vi "main 2nd.vi"() -> ()   [LabVIEW 2015]
uses:
  <vilib>/Utility/file.llb/Read From Spreadsheet File (DBL).vi
panel:
  out "From OD fit?":bool
  out "Current file num":i32
  out "ROI Width":u32
  out "ROI Height":u32
  in  "Image Dark":dbl[][](array[numeric])
  in  "Image Light":dbl[][](array[numeric])
  in  "Image Atom":dbl[][](array[numeric])
  out "Best fit parameters":dbl[](array[numeric])
  out "Fitting Results Save Path":string[](array[string])
  out "Best fit results":dbl[][](array[numeric])
  in  "Initial guess values":dbl[](array[numeric])
  in  "Latest image data":dbl[][](array[numeric])
  out "Fitting Type":u16(ring)
  out "Force Guess?":bool
  out "Aquired?":bool
  out "Process Index":i32
  out "External Trigger":bool
  out "XY图":cluster{dbl[], dbl[]}[](graph)
  out "OD Image":dbl[][](graph)
  in  "OD fit":bool
  in  "OD num":i32
  out "Fit Done":bool
  in  "Exit":bool
  out "XY图 2":cluster{dbl[], dbl[]}[](graph)
  in  "Auto Split":bool
  in  "Fit":bool
  in  "Open File":bool
  in  "Auto Fit":bool
  in  "Stop":bool
  in  "Aquire":bool
  in  "Fitting Config":bool
  in  "Camera Config":bool
  in  "Initialize":bool
  in  "Live Image Display":refnum<k7>(container)
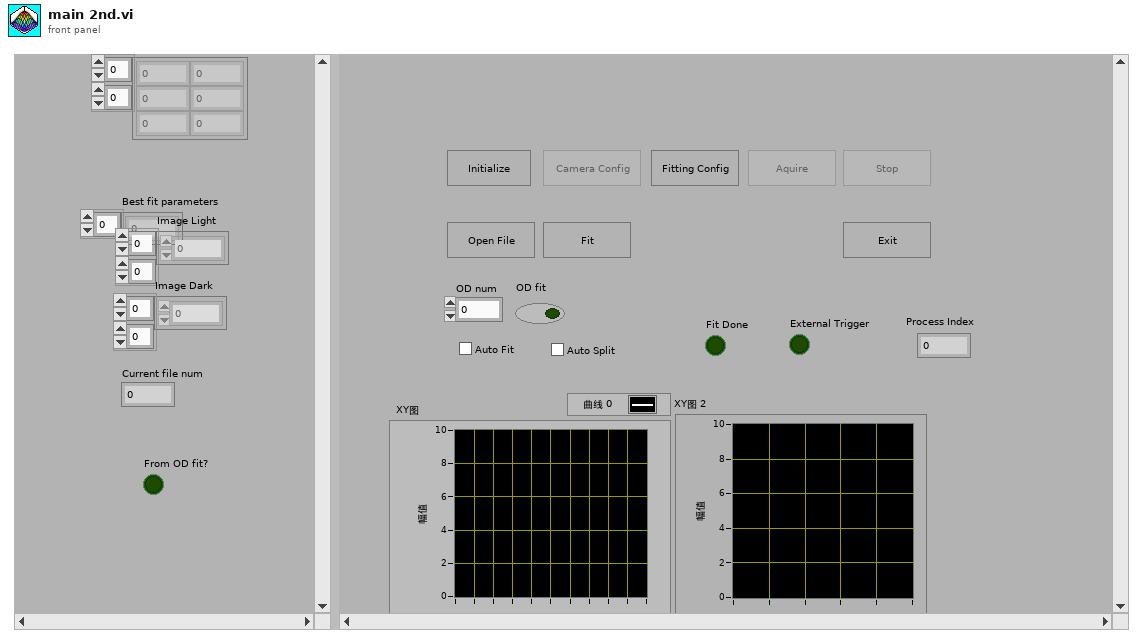
[diagram p1: front panel]
types:
  T1 = enum8{"Enabled", "Disabled", "Disabled and Grayed Out"}
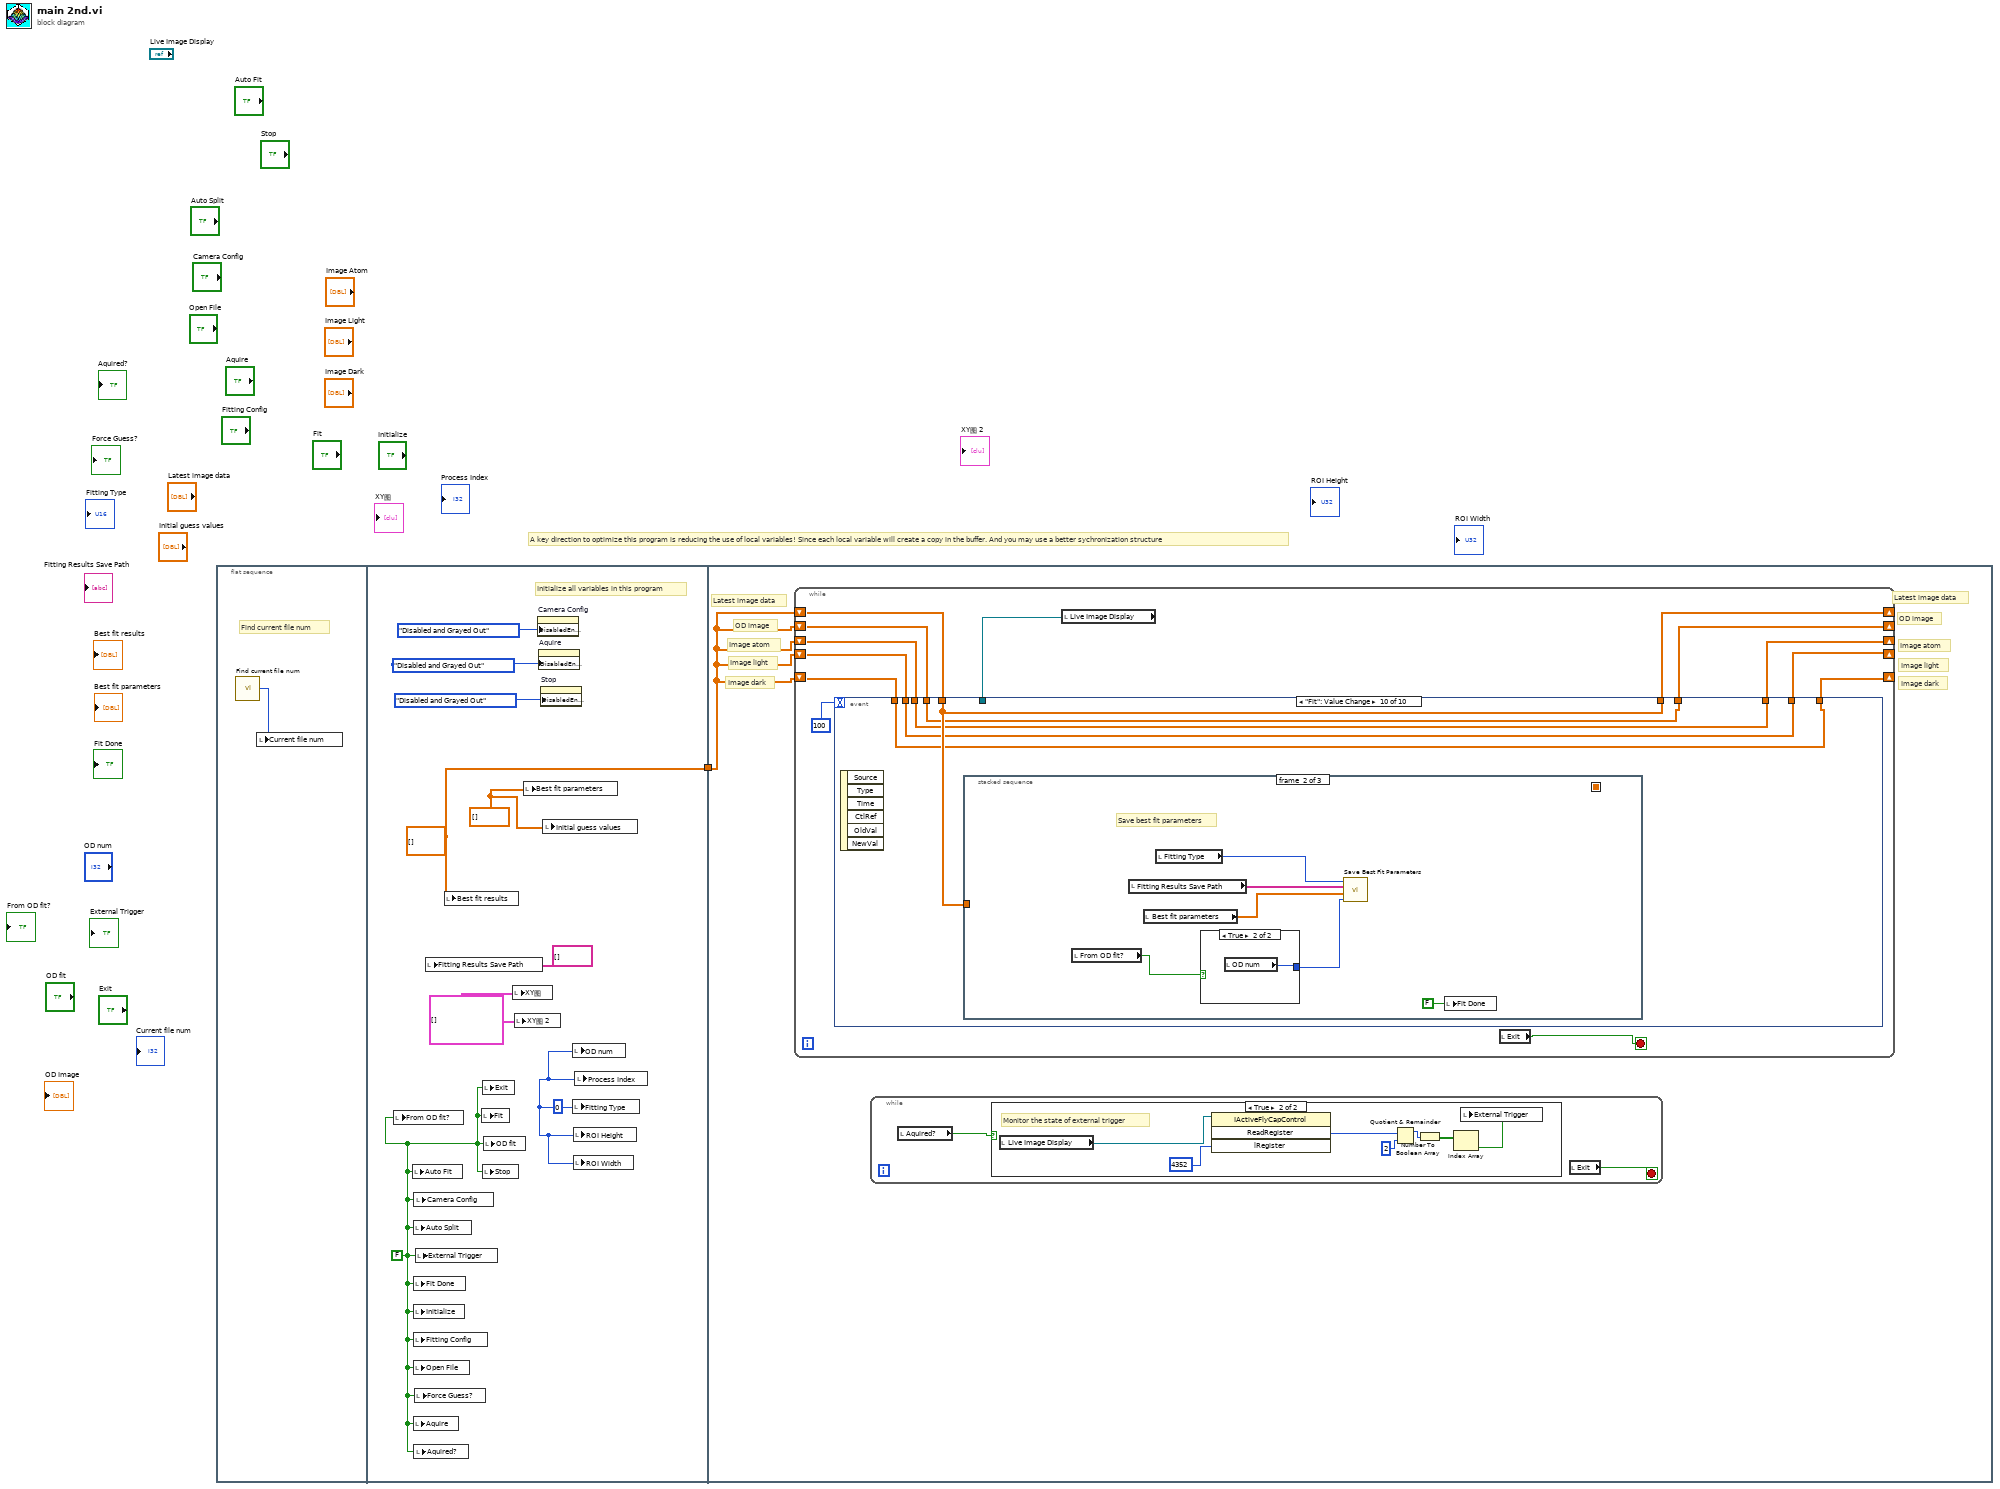
[diagram p0: block diagram]
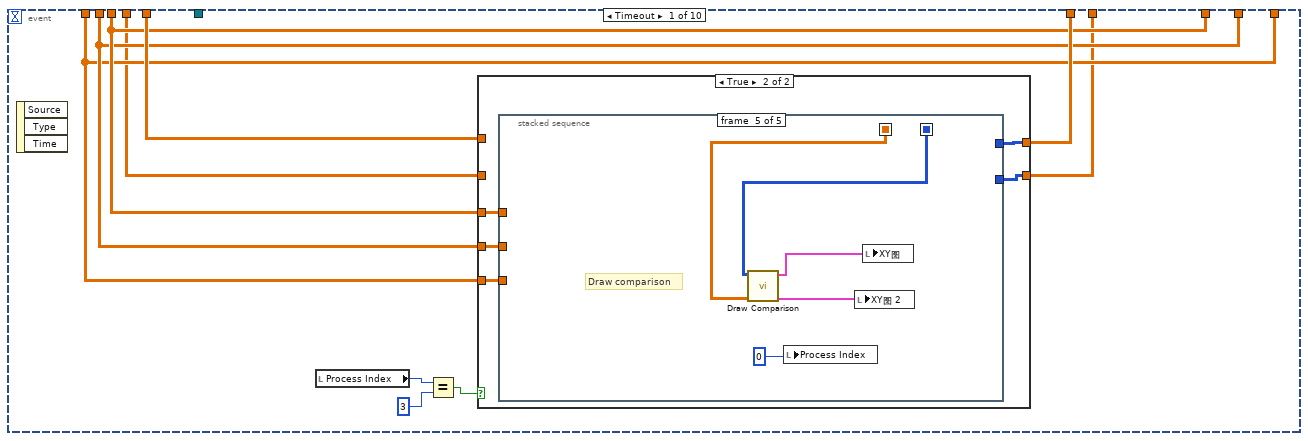
[diagram p3: hidden frame]
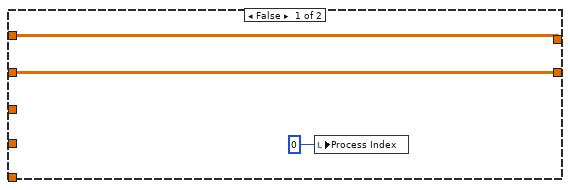
[diagram p4: hidden frame]
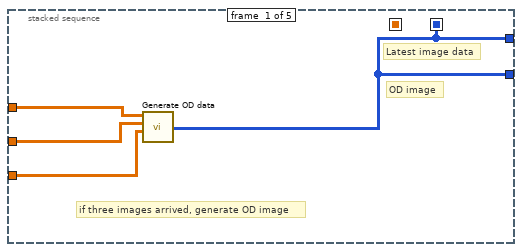
[diagram p5: hidden frame]
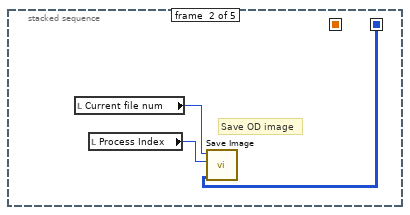
[diagram p6: hidden frame]
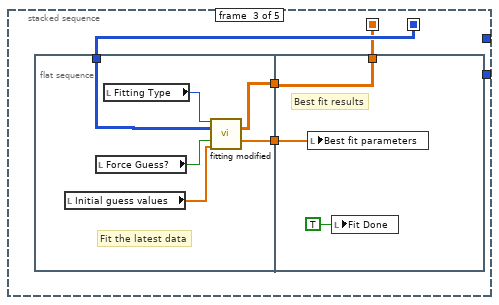
[diagram p7: hidden frame]
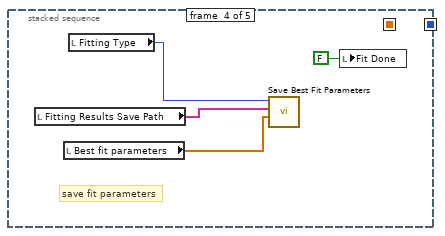
[diagram p8: hidden frame]
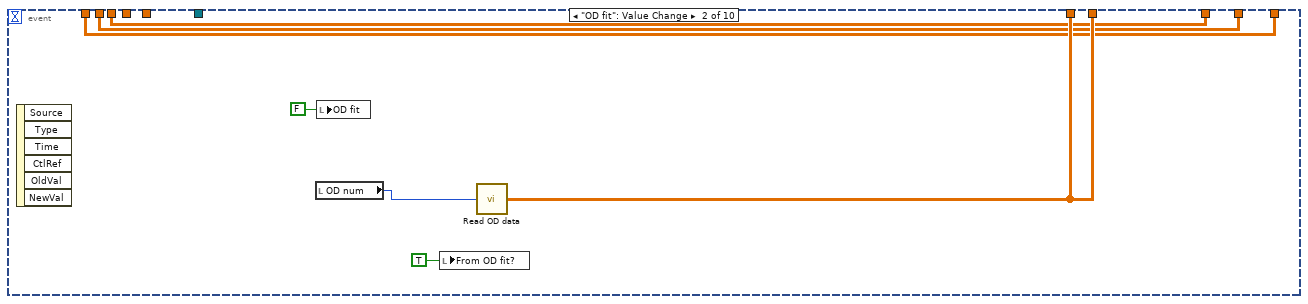
[diagram p9: hidden frame]
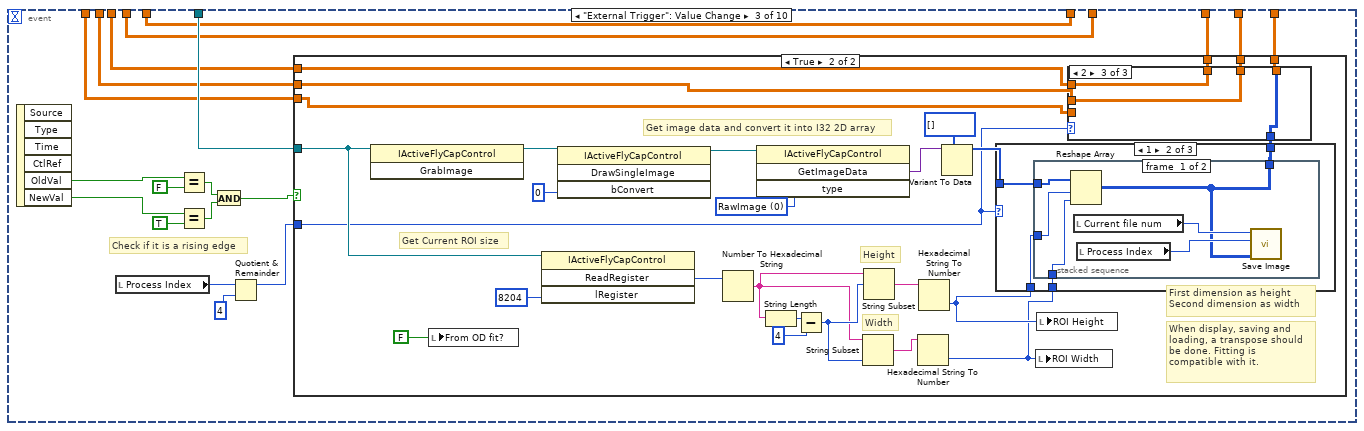
[diagram p10: hidden frame]
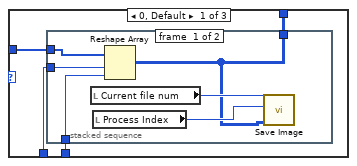
[diagram p14: hidden frame]
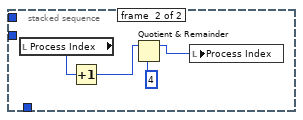
[diagram p15: hidden frame]
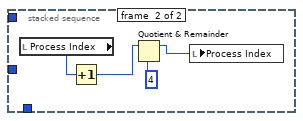
[diagram p16: hidden frame]
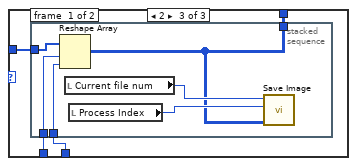
[diagram p17: hidden frame]
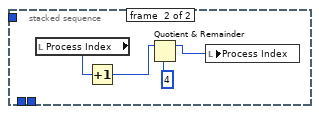
[diagram p18: hidden frame]
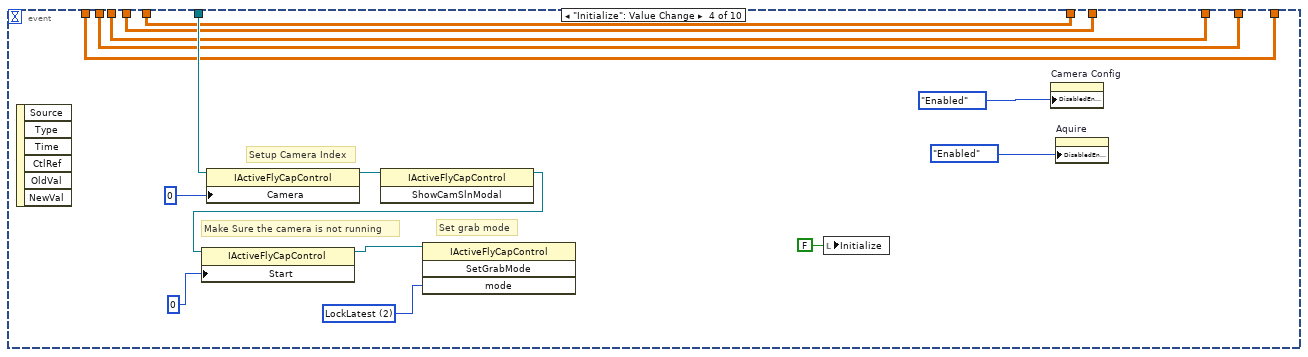
[diagram p19: hidden frame]
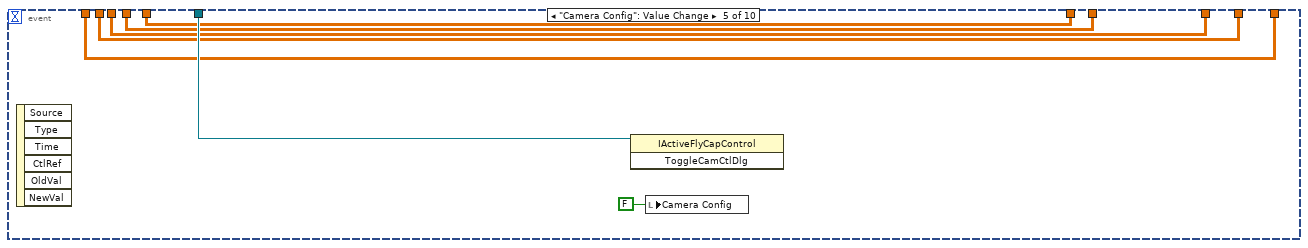
[diagram p20: hidden frame]
diagram:
  # "A key direction to optimize this program is reducing the use of local variables! Since each local variable will create a copy in the buffer. And you may use a better sychronization structure"
  n1 = flat-sequence {
    tunnel: [w5] -> w1
    tunnel: w1 -> [w12]
    frame #0 {
      # "Find current file num"
      n2 = call "Find current file num.vi"() -> ("Current File Num"=w2:u16)  [unwired: 2 in]
      n3 = local write "Current file num"(w2) -> ()
    }
    frame #1 {
      w7 = cluster{dbl[], dbl[]}[] [] ("XY图")
      w6 = 0 ("OD num")
      w5 = dbl[][] [] ("Best fit results")
      w4 = dbl[] [] ("Best fit parameters")
      w3 = FALSE ("Aquire")
      # "Initialize all variables in this program"
      n4 = local write "From OD fit?"(w3) -> ()
      n5 = local write "Auto Fit"(w3) -> ()
      n6 = local write "Auto Split"(w3) -> ()
      n7 = local write "Fit Done"(w3) -> ()
      n8 = local write "Initialize"(w3) -> ()
      n9 = local write "Fitting Config"(w3) -> ()
      n10 = local write "Open File"(w3) -> ()
      n11 = local write "Aquire"(w3) -> ()
      n12 = local write "Camera Config"(w3) -> ()
      n13 = local write "Aquired?"(w3) -> ()
      n14 = local write "Force Guess?"(w3) -> ()
      n15 = local write "External Trigger"(w3) -> ()
      n16 = local write "Fitting Results Save Path"(string[] [] ("Fitting Results Save Path")) -> ()
      n17 = local write "Best fit results"(w5) -> ()
      n18 = local write "Fit"(w3) -> ()
      n19 = local write "Exit"(w3) -> ()
      n20 = local write "Stop"(w3) -> ()
      n21 = local write "OD fit"(w3) -> ()
      n22 = local write "XY图"(w7) -> ()
      n23 = local write "XY图 2"(w7) -> ()
      n24 = local write "Best fit parameters"(w4) -> ()
      n25 = property on="Camera Config" class="Bool (strict)"("DisabledEnum"=T1."Disabled and Grayed Out" ("禁用")) -> ()  [unwired: 2 in, 2 out]
      n26 = property on="Aquire" class="Bool (strict)"("DisabledEnum"=T1."Disabled and Grayed Out" ("禁用")) -> ()  [unwired: 2 in, 2 out]
      n27 = property on="Stop" class="Bool (strict)"("DisabledEnum"=T1."Disabled and Grayed Out" ("禁用")) -> ()  [unwired: 2 in, 2 out]
      n28 = local write "Initial guess values"(w4) -> ()
      n29 = local write "OD num"(w6) -> ()
      n30 = local write "Fitting Type"(w6) -> ()
      n31 = local write "ROI Height"(w6) -> ()
      n32 = local write "ROI Width"(w6) -> ()
      n33 = local write "Process Index"(w6) -> ()
    }
    frame #2 {
      # "Image dark"
      # "Image light"
      # "Image atom"
      # "Image dark"
      # "Image light"
      # "Image atom"
      # "OD image"
      # "Latest image data"
      # "OD image"
      # "Latest image data"
      n34 = while {
        shift-right: [w31] -> _
        shift-left: w12 -> [w30]
        shift-right: [w25] -> _
        shift-left: w12 -> [w22]
        shift-right: [w24] -> _
        shift-left: w12 -> [w28]
        shift-right: [w23] -> _
        shift-left: w12 -> [w27]
        shift-right: [w29] -> _
        shift-left: w12 -> [w26]
        stop <- w32 stop-if-true
        n35 = local read "Live Image Display"() -> (w33:refnum<k7>)
        n36 = event shown="[9] \"Fit\": Value Change" {
          selector: _ -> [_ _ _ _ _ _ _ _ _ _]
          dyn-events: _ -> [_ _ _ _ _ _ _ _ _ _]
          timeout: 100 -> [_ _ _ _ _ _ _ _ _ _]
          tunnel: w33 -> [_ _ w100 w197 w210 _ _ _ _ _]
          tunnel: [w41 w86 w98 w193 w208 w215 w225 w232 w244 w256] -> w31
          tunnel: w30 -> [w40 _ w98 w193 w208 w215 w225 w232 w244 w256]
          tunnel: w22 -> [w36 _ w97 w192 w207 w214 w224 w231 w243 w255]
          tunnel: [w37 w83 w99 w189 w204 w211 w221 w228 w240 w252] -> w29
          tunnel: w28 -> [w39 w85 w96 w191 w206 w213 w223 w230 w242 w254]
          tunnel: w27 -> [w38 w84 w95 w190 w205 w212 w222 w229 w241 w253]
          tunnel: w26 -> [w37 w83 w94 w189 w204 w211 w221 w228 w240 w252]
          tunnel: [w35 w86 w97 w192 w207 w214 w224 w231 w243 w255] -> w25
          tunnel: [w39 w85 w90 w191 w206 w213 w223 w230 w242 w254] -> w24
          tunnel: [w38 w84 w89 w190 w205 w212 w222 w229 w241 w253] -> w23
          event Timeout {
            n37 = event-data() -> ()  [unwired: 1 in, 3 out]
            n38 = local read "Process Index"() -> (w44:i32)
            n39 = Equal?(x=w44, y=3) -> (x = y?=w42:bool)
            n40 = case shown="True" w42 {
              tunnel: w39 -> [_ w52]
              tunnel: w38 -> [_ w51]
              tunnel: w37 -> [_ w50]
              tunnel: [w46 w49] -> w41
              tunnel: w40 -> [w46 _]
              tunnel: w36 -> [w45 _]
              tunnel: [w45 w48] -> w35
              frame False {
                n41 = local write "Process Index"(0 ("Process Index")) -> ()
              }
              frame True {
                n42 = stacked-sequence {
                  seq-local: [w53 _ _ _ _] -> [_ w57 w61 _ w78]
                  seq-local: [_ _ w60 _ _] -> [_ _ _ _ w77]
                  tunnel: w52 -> [w56 _ _ _ _]
                  tunnel: w51 -> [w55 _ _ _ _]
                  tunnel: w50 -> [w54 _ _ _ _]
                  tunnel: [w53 _ _ _ _] -> w49
                  tunnel: [w53 _ _ _ _] -> w48
                  frame #0 {
                    # "OD image"
                    # "Latest image data"
                    # "if three images arrived, generate OD image"
                    n43 = call "Generate OD data.vi"("dark"=w54, "light"=w55, "atom"=w56) -> ("OD image"=w53:u16[][])  [unwired: 3 in]
                  }
                  frame #1 {
                    # "Save OD image"
                    n44 = local read "Current file num"() -> (w59:i32)
                    n45 = local read "Process Index"() -> (w58:i32)
                    n46 = call "Save Image.vi"("Data"=w57, "Process Index"=w58, "Current File Num"=w59) -> ()  [unwired: 9 in]
                  }
                  frame #2 {
                    n47 = flat-sequence {
                      tunnel: [w66] -> w63
                      tunnel: [w65] -> w62
                      tunnel: w61 -> [w64]
                      tunnel: w63 -> [w70]
                      tunnel: w62 -> [w72]
                      tunnel: [w70] -> w60
                      frame #0 {
                        # "Fit the latest data"
                        n48 = local read "Initial guess values"() -> (w67:dbl[])
                        n49 = local read "Force Guess?"() -> (w68:bool)
                        n50 = local read "Fitting Type"() -> (w69:u16)
                        n51 = call "fitting modified.vi"("fitting type"=w69, "2D data"=w64, "force guess?"=w68, "intial guess value"=w67) -> ("best fit"=w66:dbl[][], "best fit parameters"=w65:dbl[])  [unwired: 8 in, 2 out]
                      }
                      frame #1 {
                        # "Best fit results"
                        n52 = local write "Best fit parameters"(w72) -> ()
                        n53 = local write "Fit Done"(TRUE ("Fit Done")) -> ()
                      }
                    }
                  }
                  frame #3 {
                    # "save fit parameters"
                    n54 = local read "Fitting Results Save Path"() -> (w75:string[])
                    n55 = local read "Best fit parameters"() -> (w74:dbl[])
                    n56 = local read "Fitting Type"() -> (w76:u16)
                    n57 = call "Save Best Fit Parameters.vi"("Best Fit Parameters"=w74, "Fitting Results Save Path"=w75, "Fitting Type"=w76) -> ()  [unwired: 9 in]
                    n58 = local write "Fit Done"(FALSE ("Fit Done")) -> ()
                  }
                  frame #4 {
                    # "Draw comparison"
                    n59 = call "Draw Comparison.vi"("Best Fit"=w77, "Raw Data"=w78) -> ("Vertical Comparison"=w80:cluster{i32[], dbl[]}[], "Horizontal Comparison"=w81:cluster{i32[], dbl[]}[])  [unwired: 7 in]
                    n60 = local write "Process Index"(0 ("Process Index")) -> ()
                    n61 = local write "XY图 2"(w80) -> ()
                    n62 = local write "XY图"(w81) -> ()
                  }
                }
              }
            }
          }
          event "OD fit": Value Change {
            n63 = event-data() -> ()  [unwired: 1 in, 6 out]
            n64 = local read "OD num"() -> (w87:i32)
            n65 = local write "OD fit"(FALSE ("OD fit")) -> ()
            n66 = local write "From OD fit?"(TRUE ("From OD fit?")) -> ()
            n67 = call "Read OD data.vi"("OD num"=w87) -> ("OD data"=w86:dbl[][])  [unwired: 4 in]
          }
          event "External Trigger": Value Change {
            # "Check if it is a rising edge"
            n68 = event-data() -> ("OldVal"=w105:bool, "NewVal"=w104:bool)  [unwired: 1 in, 4 out]
            n69 = local read "Process Index"() -> (w92:i32)
            n70 = Equal?(x=w105, y=FALSE) -> (x = y?=w107:bool)
            n71 = Equal?(x=w104, y=TRUE) -> (x = y?=w106:bool)
            n72 = And(x=w107, y=w106) -> (x .and. y?=w101:bool)
            n73 = Quotient & Remainder(x=w92, y=4) -> (x-y*floor(x/y)=w91:i32)  [unwired: 1 out]
            n74 = case shown="True" w101 {
              tunnel: w100 -> [_ w133]
              tunnel: [w108 w114] -> w99
              tunnel: w96 -> [w110 w118]
              tunnel: w95 -> [w109 w117]
              tunnel: w94 -> [w108 w116]
              tunnel: w91 -> [_ w119]
              tunnel: [w110 w112] -> w90
              tunnel: [w109 w115] -> w89
              frame False {
              }
              frame True {
                w134 = 0 items=["RawImage", "ColorProcessedImage"] ("type")
                # "Get image data and convert it into I32 2D array"
                # "When display, saving and \nloading, a transpose should\nbe done. Fitting is \ncompatible with it."
                # "First dimension as height\nSecond dimension as width"
                # "Width"
                # "Height"
                # "Get Current ROI size"
                n75 = invoke class="IActiveFlyCapControl" method="GrabImage"(reference=w133) -> (reference out=w137:refnum<k7>)  [unwired: 2 in, 2 out]
                n76 = local write "From OD fit?"(FALSE ("From OD fit?")) -> ()
                n77 = invoke class="IActiveFlyCapControl" method="ReadRegister"(reference=w133, "lRegister"=u32 8204) -> ("ReadRegister"=w130:u32)  [unwired: 2 in, 3 out]
                n78 = invoke class="IActiveFlyCapControl" method="DrawSingleImage"(reference=w137, "bConvert"=0) -> (reference out=w136:refnum<k7>)  [unwired: 2 in, 3 out]
                n79 = Number To Hexadecimal String(2:w130) -> (0:w126:string)  [unwired: 1 in]
                n80 = invoke class="IActiveFlyCapControl" method="GetImageData"(reference=w136, "type"=w134) -> ("GetImageData"=w131:variant)  [unwired: 2 in, 3 out]
                n81 = String Length(string=w126) -> (length=w129:i32)
                n82 = Subtract(x=w129, y=4) -> (x-y=w127:i32)
                n83 = String Subset(string=w126, length (rest)=w127) -> (substring=w123:string)  [unwired: 1 in]
                n84 = String Subset(string=w126, offset (0)=w127) -> (substring=w124:string)  [unwired: 1 in]
                n85 = Hexadecimal String To Number(string=w123) -> (number=w120:u32)  [unwired: 2 in, 1 out]
                n86 = Hexadecimal String To Number(string=w124) -> (number=w121:u32)  [unwired: 2 in, 1 out]
                n87 = Variant To Data(type=i32[] [], Variant=w131) -> (data=w122:i32[])  [unwired: 1 in, 1 out]
                n88 = case shown="1" w119 {
                  tunnel: w122 -> [w150 w164 w178]
                  tunnel: w121 -> [w149 w163 w177]
                  tunnel: w120 -> [w148 w162 w176]
                  tunnel: [w147 w161 w175] -> w113
                  frame 0, Default {
                    n89 = stacked-sequence {
                      tunnel: w150 -> [w154 _]
                      tunnel: w149 -> [w153 _]
                      tunnel: w148 -> [w152 _]
                      tunnel: [w151 _] -> w147
                      frame #0 {
                        n90 = local read "Current file num"() -> (w156:i32)
                        n91 = local read "Process Index"() -> (w155:i32)
                        n92 = Reshape Array(w154, w153, w152) -> (w151:i32[][])
                        n93 = call "Save Image.vi"("Data"=w151, "Process Index"=w155, "Current File Num"=w156) -> ()  [unwired: 9 in]
                      }
                      frame #1 {
                        n94 = local read "Process Index"() -> (w160:i32)
                        n95 = Increment(x=w160) -> (x+1=w159:i32)
                        n96 = Quotient & Remainder(x=w159, y=4) -> (x-y*floor(x/y)=w157:i32)  [unwired: 1 out]
                        n97 = local write "Process Index"(w157) -> ()
                      }
                    }
                  }
                  frame 1 {
                    n98 = stacked-sequence {
                      tunnel: w164 -> [w166 _]
                      tunnel: w163 -> [w168 _]
                      tunnel: w162 -> [w167 _]
                      tunnel: [w165 _] -> w161
                      frame #0 {
                        n99 = Reshape Array(w166, w168, w167) -> (w165:i32[][])
                        n100 = local read "Current file num"() -> (w170:i32)
                        n101 = local read "Process Index"() -> (w169:i32)
                        n102 = call "Save Image.vi"("Data"=w165, "Process Index"=w169, "Current File Num"=w170) -> ()  [unwired: 9 in]
                      }
                      frame #1 {
                        n103 = local read "Process Index"() -> (w174:i32)
                        n104 = Increment(x=w174) -> (x+1=w173:i32)
                        n105 = Quotient & Remainder(x=w173, y=4) -> (x-y*floor(x/y)=w171:i32)  [unwired: 1 out]
                        n106 = local write "Process Index"(w171) -> ()
                      }
                    }
                  }
                  frame 2 {
                    n107 = stacked-sequence {
                      tunnel: w178 -> [w182 _]
                      tunnel: w177 -> [w181 _]
                      tunnel: w176 -> [w180 _]
                      tunnel: [w179 _] -> w175
                      frame #0 {
                        n108 = Reshape Array(w182, w181, w180) -> (w179:i32[][])
                        n109 = local read "Current file num"() -> (w184:i32)
                        n110 = local read "Process Index"() -> (w183:i32)
                        n111 = call "Save Image.vi"("Data"=w179, "Process Index"=w183, "Current File Num"=w184) -> ()  [unwired: 9 in]
                      }
                      frame #1 {
                        n112 = local read "Process Index"() -> (w188:i32)
                        n113 = Increment(x=w188) -> (x+1=w187:i32)
                        n114 = Quotient & Remainder(x=w187, y=4) -> (x-y*floor(x/y)=w185:i32)  [unwired: 1 out]
                        n115 = local write "Process Index"(w185) -> ()
                      }
                    }
                  }
                }
                n116 = local write "ROI Width"(w120) -> ()
                n117 = local write "ROI Height"(w121) -> ()
                n118 = case shown="2" w119 {
                  tunnel: w118 -> [_ w143 w146]
                  tunnel: w117 -> [w140 _ w145]
                  tunnel: w116 -> [w139 w142 _]
                  tunnel: [w140 w141 w145] -> w115
                  tunnel: [w139 w142 w144] -> w114
                  tunnel: w113 -> [w138 w141 w144]
                  tunnel: [w138 w143 w146] -> w112
                  frame 0, Default {
                  }
                  frame 1 {
                  }
                  frame 2 {
                  }
                }
              }
            }
          }
          event "Initialize": Value Change {
            w201 = 2 items=["FreeRunning", "LockNext", "LockLatest"] ("mode")
            # "Setup Camera Index"
            # "Set grab mode"
            # "Make Sure the camera is not running"
            n119 = event-data() -> ()  [unwired: 1 in, 6 out]
            n120 = property class="IActiveFlyCapControl"(reference=w197, "Camera"=0 ("Start")) -> (reference out=w200:refnum<k7>)  [unwired: 1 in, 1 out]
            n121 = invoke class="IActiveFlyCapControl" method="ShowCamSlnModal"(reference=w200) -> (reference out=w196:refnum<k7>)  [unwired: 2 in, 2 out]
            n122 = property class="IActiveFlyCapControl"(reference=w196, "Start"=0 ("Camera")) -> (reference out=w195:refnum<k7>)  [unwired: 1 in, 1 out]
            n123 = invoke class="IActiveFlyCapControl" method="SetGrabMode"(reference=w195, "mode"=w201) -> ()  [unwired: 2 in, 4 out]
            n124 = local write "Initialize"(FALSE ("Initialize")) -> ()
            n125 = property on="Camera Config" class="Bool (strict)"("DisabledEnum"=T1."Enabled" ("禁用")) -> ()  [unwired: 2 in, 2 out]
            n126 = property on="Aquire" class="Bool (strict)"("DisabledEnum"=T1."Enabled" ("禁用")) -> ()  [unwired: 2 in, 2 out]
          }
          event "Camera Config": Value Change {
            n127 = event-data() -> ()  [unwired: 1 in, 6 out]
            n128 = invoke class="IActiveFlyCapControl" method="ToggleCamCtlDlg"(reference=w210) -> ()  [unwired: 2 in, 3 out]
            n129 = local write "Camera Config"(FALSE ("Camera Config")) -> ()
          }
          event "Fitting Config": Value Change {
            # "pump out fitting config. and transfer parameters"
            n130 = event-data() -> ()  [unwired: 1 in, 6 out]
            n131 = call "Fitting Configuration.vi"() -> ("intial guess"=w216:dbl[], "Force Guess？"=w217:bool, "Fitting Type"=w219:u16, "Fitting Results Save Path"=w218:string[])  [unwired: 5 in]
            n132 = local write "Fitting Results Save Path"(w218) -> ()
            n133 = local write "Fitting Type"(w219) -> ()
            n134 = local write "Fitting Config"(FALSE ("Fitting Config")) -> ()
            n135 = local write "Initial guess values"(w216) -> ()
            n136 = local write "Force Guess?"(w217) -> ()
          }
          event "Open File": Value Change {
            n137 = event-data() -> ()  [unwired: 1 in, 6 out]
            n138 = call-poly <vilib>:"Read From Spreadsheet File.vi"() -> ("all rows"=w226:dbl[][])  [unwired: 7 in, 4 out]
            n139 = local write "Open File"(FALSE ("Open File")) -> ()
            n140 = local write "Latest image data"(w226) -> ()
            n141 = local write "OD Image"(w226) -> ()
          }
          event "Aquire": Value Change {
            # "Start the camera"
            n142 = event-data() -> ()  [unwired: 1 in, 6 out]
            n143 = property on="Aquire" class="Bool (strict)"("DisabledEnum"=T1."Disabled and Grayed Out" ("禁用")) -> ()  [unwired: 2 in, 2 out]
            n144 = property on="Stop" class="Bool (strict)"("DisabledEnum"=T1."Enabled" ("禁用")) -> ()  [unwired: 2 in, 2 out]
            n145 = property on="Camera Config" class="Bool (strict)"("DisabledEnum"=T1."Disabled and Grayed Out" ("禁用")) -> ()  [unwired: 2 in, 2 out]
            n146 = local read "Live Image Display"() -> (w234:refnum<k7>)
            n147 = local write "Aquire"(FALSE ("Initialize")) -> ()
            n148 = local write "Aquired?"(TRUE ("Aquired?")) -> ()
            n149 = property class="IActiveFlyCapControl"(reference=w234, "Start"=1) -> ()  [unwired: 1 in, 2 out]
          }
          event "Stop": Value Change {
            # "stop the camera"
            n150 = event-data() -> ()  [unwired: 1 in, 6 out]
            n151 = property on="Stop" class="Bool (strict)"("DisabledEnum"=T1."Disabled and Grayed Out" ("禁用")) -> ()  [unwired: 2 in, 2 out]
            n152 = property on="Aquire" class="Bool (strict)"("DisabledEnum"=T1."Disabled and Grayed Out" ("禁用")) -> ()  [unwired: 2 in, 2 out]
            n153 = local read "Live Image Display"() -> (w247:refnum<k7>)
            n154 = local write "Stop"(FALSE ("Initialize")) -> ()
            n155 = property class="IActiveFlyCapControl"(reference=w247, "Start"=0) -> (reference out=w246:refnum<k7>)  [unwired: 1 in, 1 out]
            n156 = local write "Aquired?"(FALSE ("Aquired?")) -> ()
            n157 = local write "Live Image Display"(w246) -> ()
          }
          event "Fit": Value Change {
            n158 = event-data() -> ()  [unwired: 1 in, 6 out]
            n159 = stacked-sequence {
              seq-local: [w257 _ _] -> [_ _ w280]
              tunnel: w256 -> [w258 _ w281]
              frame #0 {
                n160 = flat-sequence {
                  tunnel: [w263] -> w260
                  tunnel: [w262] -> w259
                  tunnel: w258 -> [w261]
                  tunnel: w260 -> [w267]
                  tunnel: w259 -> [w270]
                  tunnel: [w267] -> w257
                  frame #0 {
                    # "Fit the latest data"
                    n161 = local read "Initial guess values"() -> (w265:dbl[])
                    n162 = local read "Force Guess?"() -> (w266:bool)
                    n163 = local read "Fitting Type"() -> (w264:u16)
                    n164 = call "fitting modified.vi"("fitting type"=w264, "2D data"=w261, "force guess?"=w266, "intial guess value"=w265) -> ("best fit"=w263:dbl[][], "best fit parameters"=w262:dbl[])  [unwired: 8 in, 2 out]
                  }
                  frame #1 {
                    # "Best fit results"
                    n165 = local write "Fit"(FALSE ("Fit")) -> ()
                    n166 = local write "Best fit parameters"(w270) -> ()
                    n167 = local write "Fit Done"(TRUE ("Fit Done")) -> ()
                  }
                }
              }
              frame #1 {
                # "Save best fit parameters"
                n168 = local read "From OD fit?"() -> (w272:bool)
                n169 = local read "Fitting Results Save Path"() -> (w274:string[])
                n170 = local read "Best fit parameters"() -> (w273:dbl[])
                n171 = local read "Fitting Type"() -> (w275:u16)
                n172 = case shown="True" w272 {
                  tunnel: [w277 w278] -> w271
                  frame False {
                    n173 = local read "Current file num"() -> (w277:i32)
                  }
                  frame True {
                    n174 = local read "OD num"() -> (w278:i32)
                  }
                }
                n175 = call "Save Best Fit Parameters.vi"("Current File Num"=w271, "Best Fit Parameters"=w273, "Fitting Results Save Path"=w274, "Fitting Type"=w275) -> ()  [unwired: 8 in]
                n176 = local write "Fit Done"(FALSE ("Fit Done")) -> ()
              }
              frame #2 {
                # "Draw Comparison"
                n177 = local write "From OD fit?"(FALSE ("From OD fit?")) -> ()
                n178 = local write "Fit"(FALSE ("Initialize")) -> ()
                n179 = call "Draw Comparison.vi"("Best Fit"=w280, "Raw Data"=w281) -> ("Vertical Comparison"=w283:cluster{i32[], dbl[]}[], "Horizontal Comparison"=w284:cluster{i32[], dbl[]}[])  [unwired: 7 in]
                n180 = local write "XY图 2"(w283) -> ()
                n181 = local write "XY图"(w284) -> ()
              }
            }
          }
        }
        n182 = local read "Exit"() -> (w32:bool)
      }
      n183 = while {
        stop <- w14 stop-if-true
        n184 = local read "Aquired?"() -> (w13:bool)
        n185 = case shown="True" w13 {
          frame False {
          }
          frame True {
            # "Monitor the state of external trigger"
            n186 = local read "Live Image Display"() -> (w21:refnum<k7>)
            n187 = invoke class="IActiveFlyCapControl" method="ReadRegister"(reference=w21, "lRegister"=u32 4352) -> ("ReadRegister"=w19:u32)  [unwired: 2 in, 3 out]
            n188 = Quotient & Remainder(x=w19, y=u32 2) -> (x-y*floor(x/y)=w17:u32)  [unwired: 1 out]
            n189 = Number To Boolean Array(number=w17) -> (Boolean array=w16:bool[])
            n190 = Index Array(array=w16) -> (element=w15:bool)  [unwired: 1 in]
            n191 = local write "External Trigger"(w15) -> ()
          }
        }
        n192 = local read "Exit"() -> (w14:bool)
      }
    }
  }
